vi "GUI_Frog_HPD_Version 2.0.vi"() -> ()   [LabVIEW 2020]
uses:
  Shared/GUI_Template/GUI_master/tcp_new_data_event.ctl
  Shared/GUI_Template/GUI_master/tcp new data cluster.ctl
  GUI_Cameras/color tables/image color table presets.ctl
  <vilib>/vision/Image Controls.llb/IMAQ Image.ctl
  <vilib>/vision/NI_Vision_Development_Module.lvlib
panel:
  in  "Color table":T1=enum."Binary"
  out "Time":sgl[](graph)
  out "Spectrum":sgl[](graph)
  out "tcp data event 2":T2
  out "Tank":dbl(slide) scale=0.0..255.0 scale format="%#_6p"
  out "131":T3(plugin-control) caption="Spatial Image"
  out "525":T3(plugin-control) caption="FROG Trace"
  out "error out":errorcluster
  in  "Clear":bool
  in  "UDP error message":string
  in  "Refresh Button":bool
  in  "Tab Control":T4(tab)
  in  "exposure::1":dbl=0.001 caption="Exposure" min=5.0 max=10000.0 format="%_4p"
  out "frogerrorfinal::1":dbl caption="Frog Error (<1% OK)" min=0.0 max=500.0
  in  "cameraselect::1":enum16{"temporal CAM", "spatial CAM"}(ring) caption="Select Camera"
  in  "triggermode::1":bool caption="Blank Button"
  in  "Select device":string(combo)="FrogHPD"
  out "GUIdevice 1":string="FrogHPD"
  out "element":string
  out "Application:Command Line Arguments":string[](array[string])
  out "max counts":cluster{dbl[], dbl[]}(graph)
  out "mean counts":cluster{dbl[], dbl[]}(graph)
  out "Fourier analyzed data":T5
  in  "fourier":bool
  out "SpatialImage::1":T3(plugin-control) caption="Spatial Image"
  out "frogTrace::1":T3(plugin-control) caption="FROG Trace"
  in  "insert tag":bool=TRUE
  in  "stop":bool
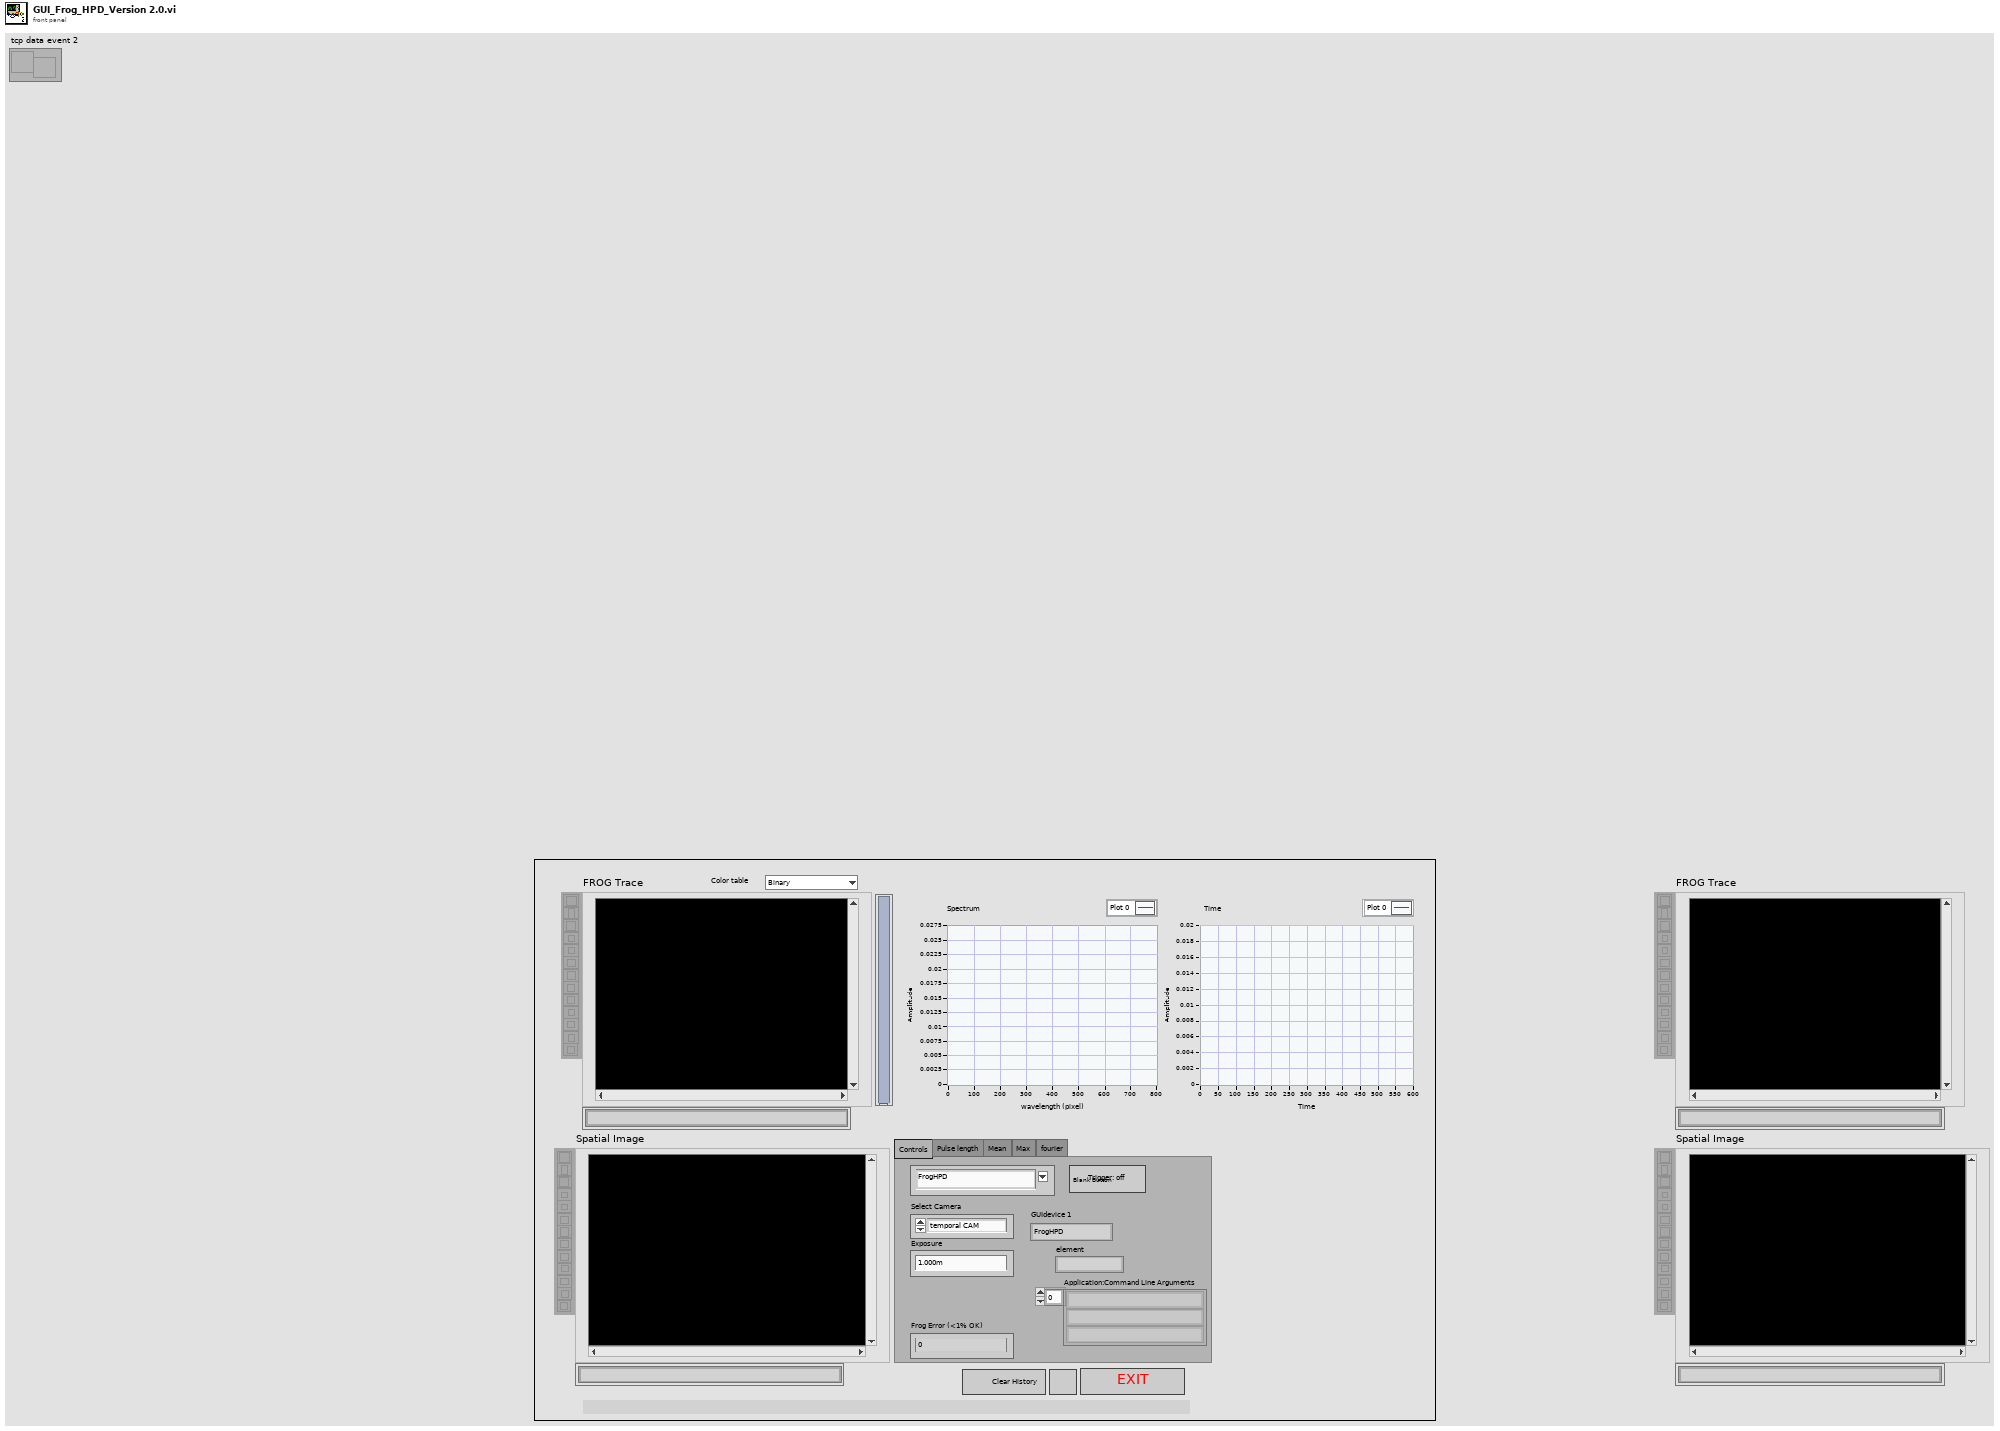
[diagram p1: front panel]
types:
  T1 = typedef "image color table presets.ctl" = enum16{"Greyscale", "Binary", "Gradient", "Rainbow", "Temperature", "enhance low", "blue yellow red", "BYR enhance low", "white blue yellow", "BWR enhance low", "make a new one"}
  T2 = typedef "tcp_new_data_event.ctl" = refnum<user-event>
  T3 = typedef "IMAQ Image.ctl" = refnum<image>
  T4 = enum32{"Controls", "Pulse length", "Mean", "Max", "fourier"}
  T5 = cluster{"Amplitude":dbl, "Frequency":dbl, "period":dbl}
  T6 = enum32{"invalid app kind", "Development System", "Run Time System", "Student Edition", "Embedded LabVIEW", "Evaluation", "Custom"}
  T7 = typedef "tcp new data cluster.ctl" = cluster{"EventEnum":enum16{"new data", "connection status update"}, "Device name":string}
  T8 = enum32{"Invalid", "Standard", "Closed", "Hidden", "Minimized", "Maximized"}
  T9 = cluster{"Left":i32, "Top":i32, "Right":i32, "Bottom":i32}
  T10 = cluster{"Core":cluster{"Current VI Reference":refnum<vi>, "Close Panel on Exit?":bool}, "Your Boolean data":bool, "Your string data":string, "SuperGUI":cluster{"STOP queue":refnum<queue>, "SuperGUI ref":refnum<vi>, "event reg":refnum<event-registration>}, "Images":cluster{"frogTrace::1":T3, "retrievedFrogTrace::1":T3, "SpatialImage::1":T3, "rotated_Temporal":T3, "rotated_Spatial":T3}}
  T11 = cluster{"frogTrace::1":T3, "retrievedFrogTrace::1":T3, "SpatialImage::1":T3, "rotated_Temporal":T3, "rotated_Spatial":T3}
  T12 = cluster{"STOP queue":refnum<queue>, "SuperGUI ref":refnum<vi>, "event reg":refnum<event-registration>}
  T13 = cluster{"Current VI Reference":refnum<vi>, "Close Panel on Exit?":bool}
  T14 = cluster{"histogram":u32[], "Minimal Value":sgl, "Maximal Value":sgl, "Starting Value":sgl, "Interval Width":sgl, "Mean Value":sgl, "Standard  Variation":sgl, "Area (pixels)":i32}
  T15 = typedef "Image Type" = u32
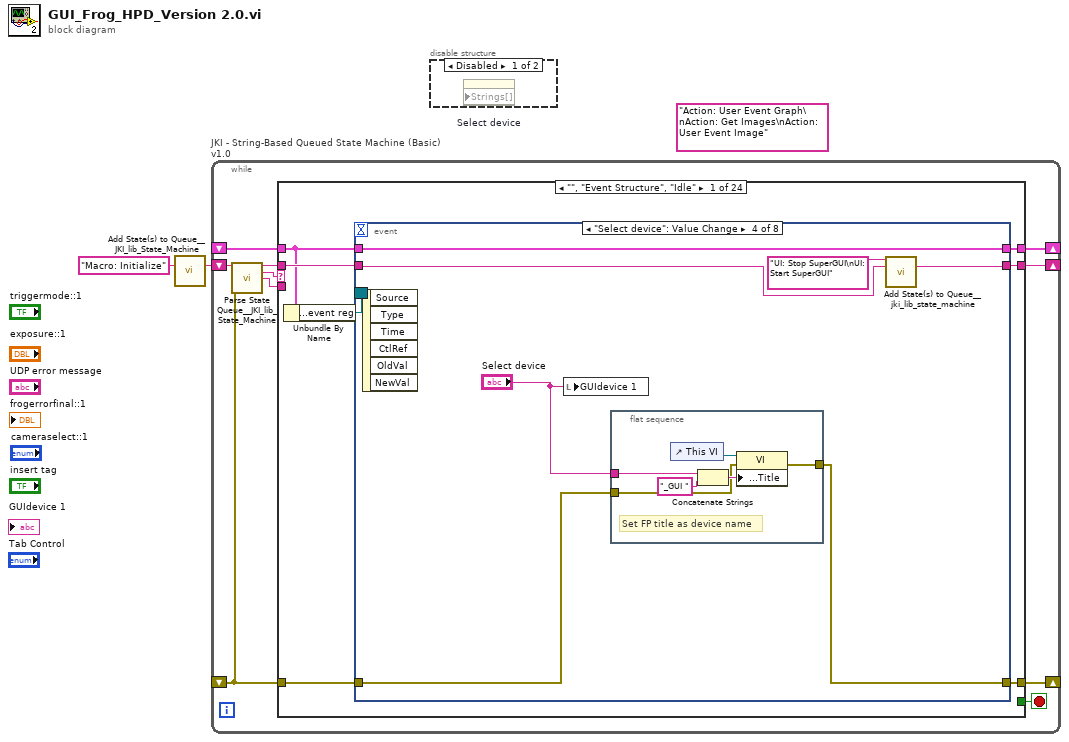
[diagram p0: block diagram]
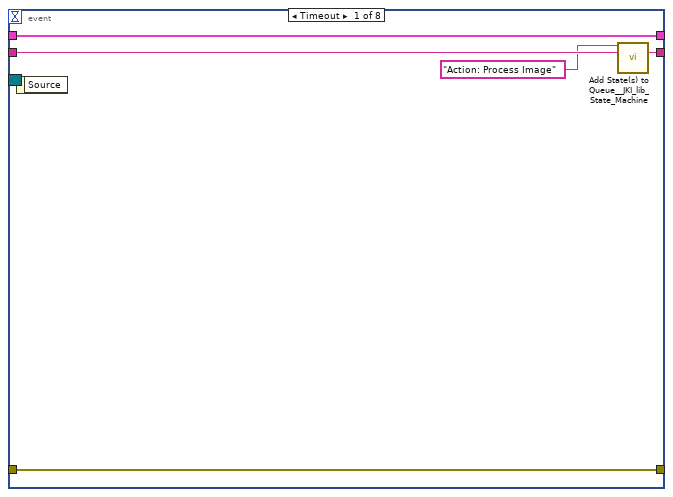
[diagram p3: hidden frame]
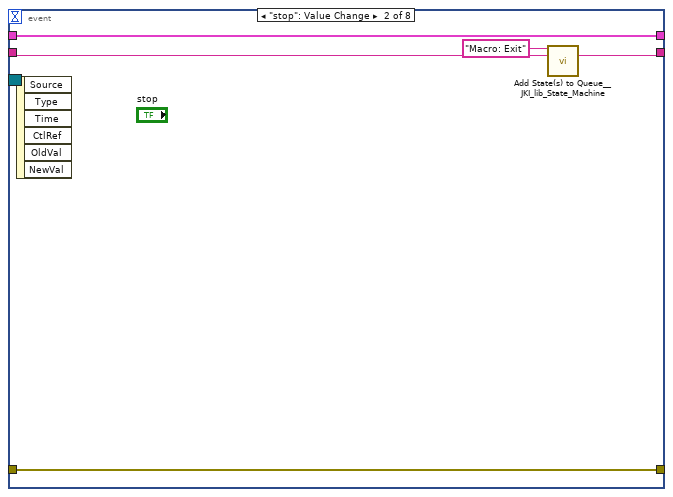
[diagram p4: hidden frame]
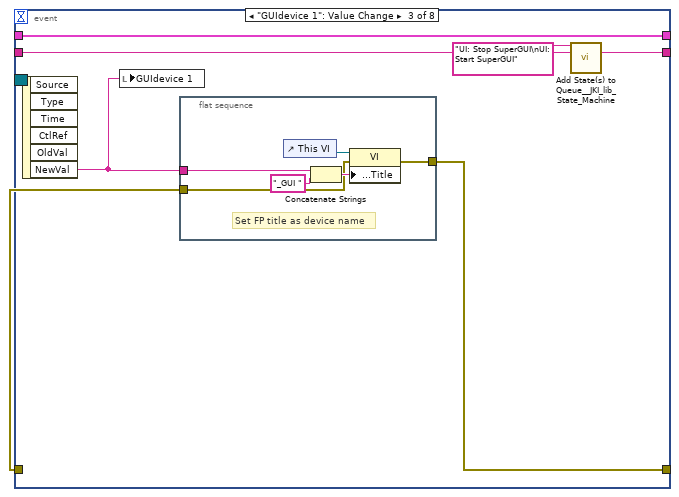
[diagram p5: hidden frame]
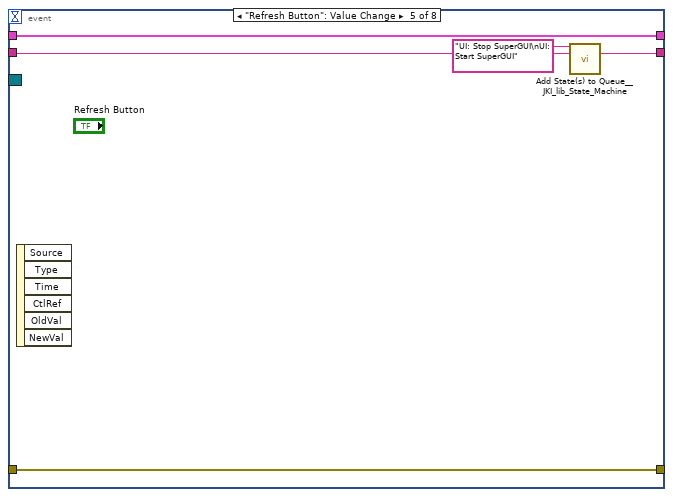
[diagram p6: hidden frame]
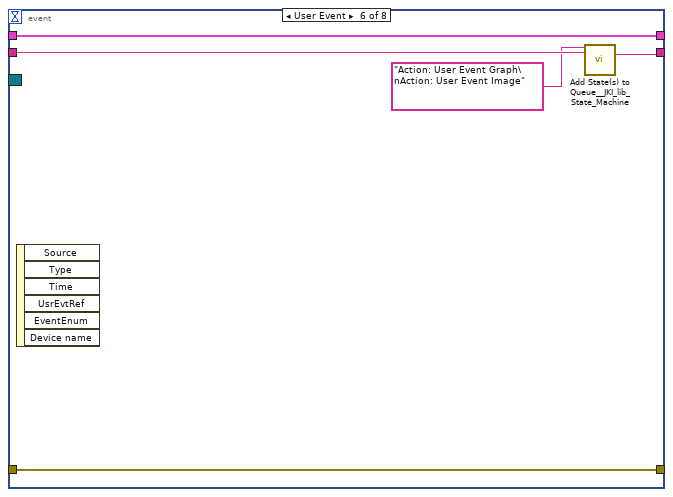
[diagram p7: hidden frame]
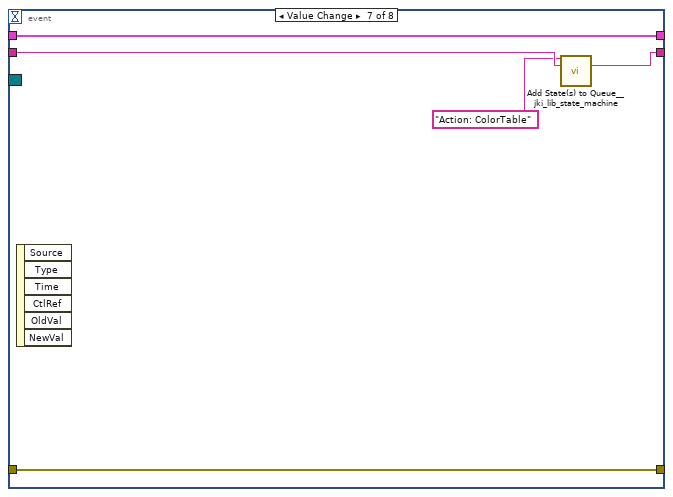
[diagram p8: hidden frame]
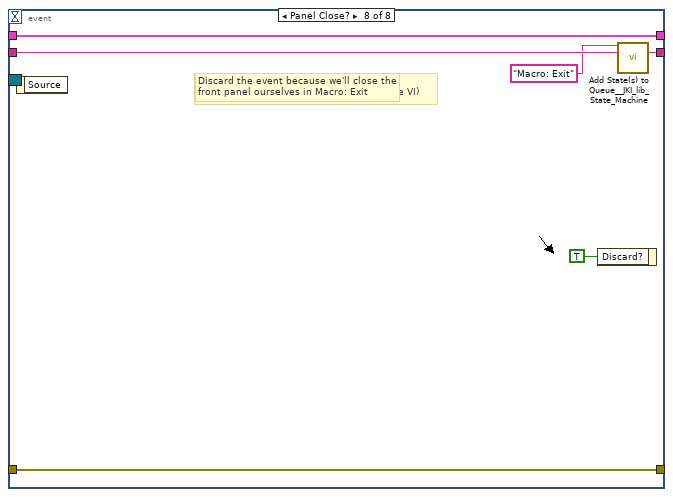
[diagram p9: hidden frame]
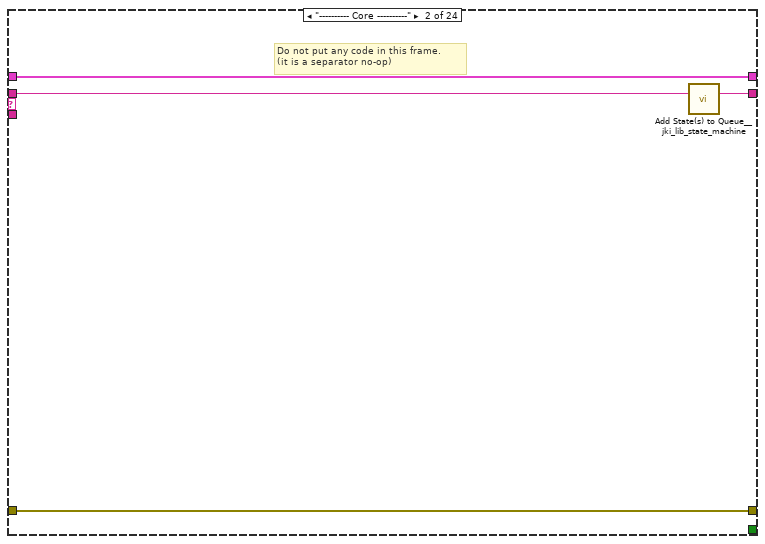
[diagram p10: hidden frame]
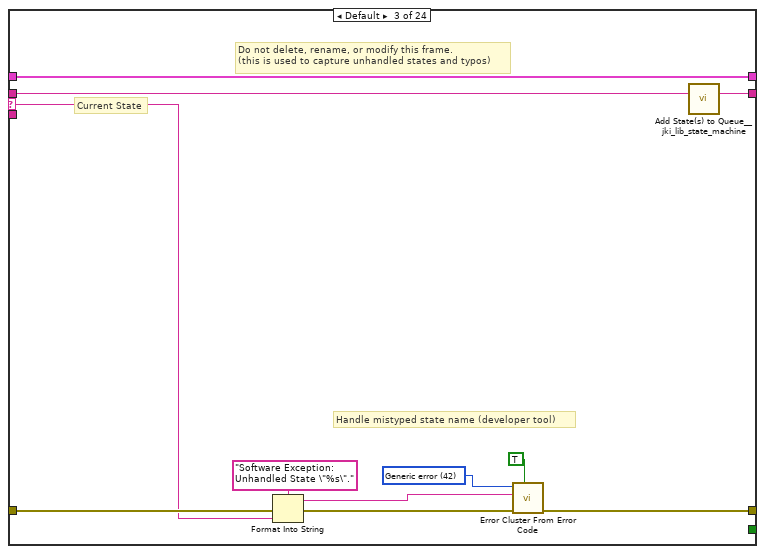
[diagram p11: hidden frame]
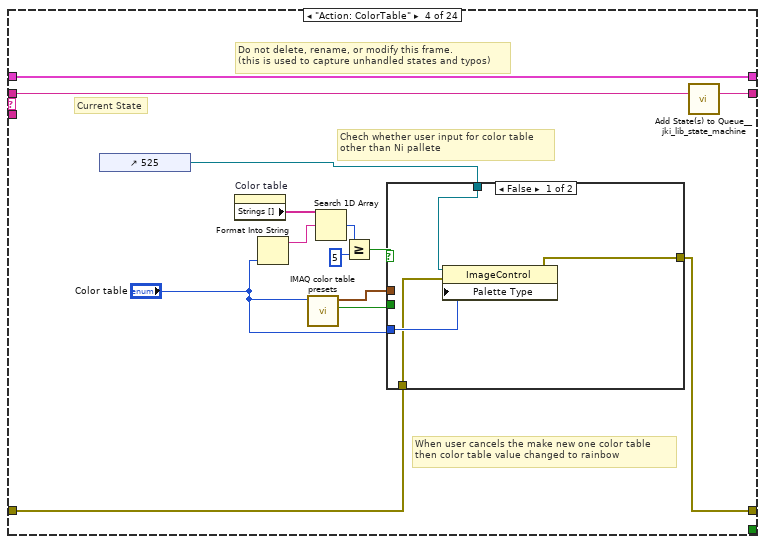
[diagram p12: hidden frame]
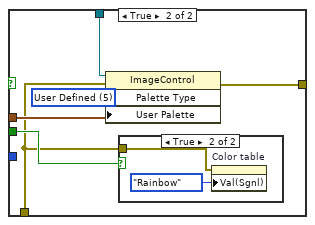
[diagram p13: hidden frame]
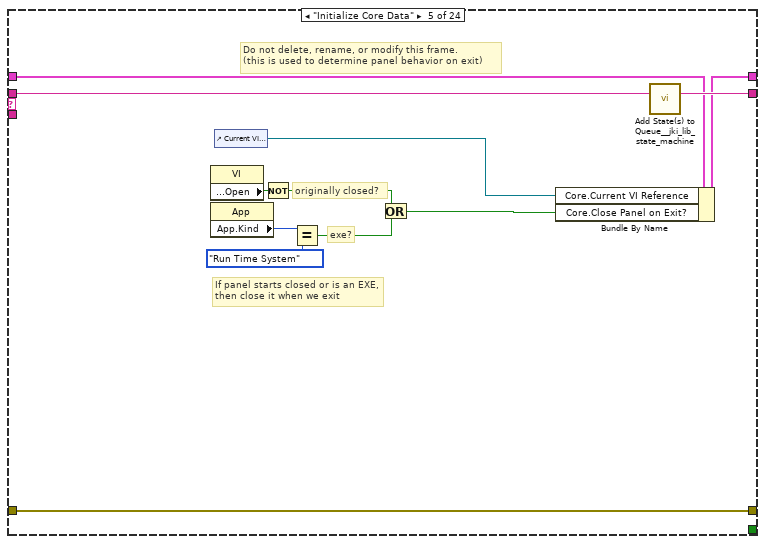
[diagram p15: hidden frame]
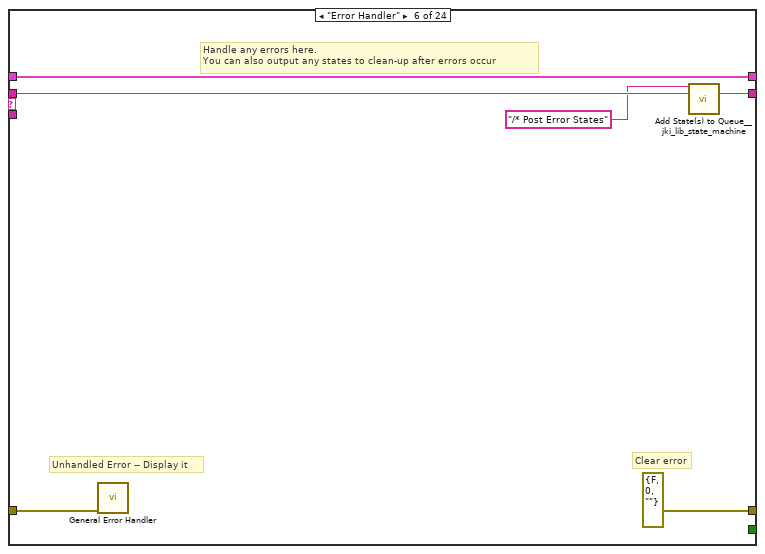
[diagram p16: hidden frame]
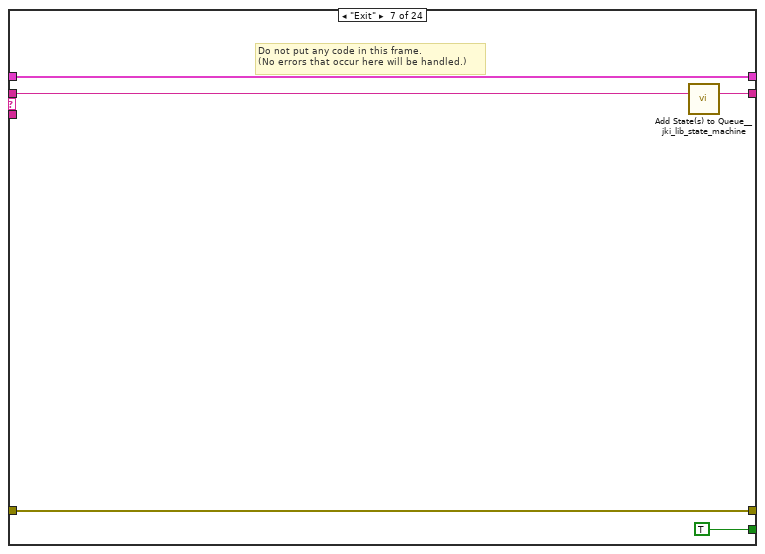
[diagram p17: hidden frame]
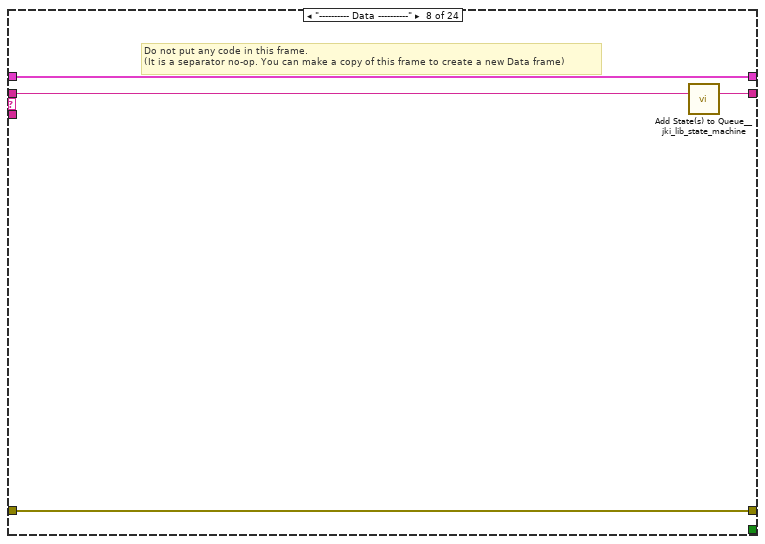
[diagram p18: hidden frame]
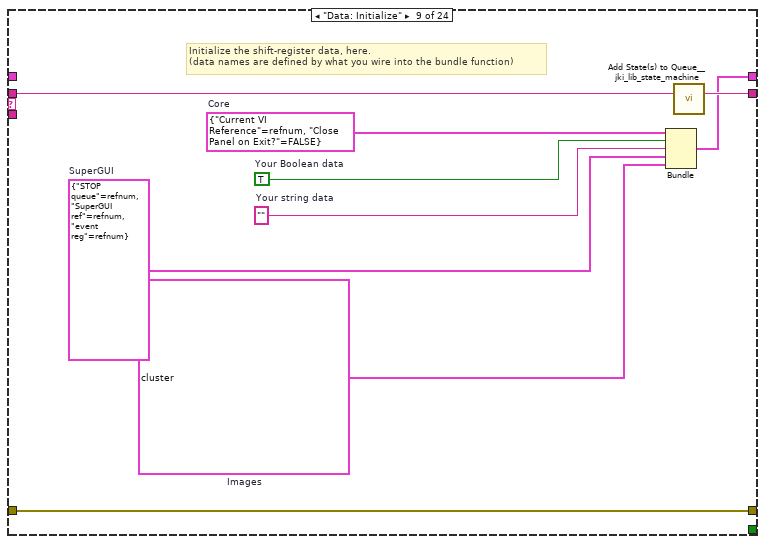
[diagram p19: hidden frame]
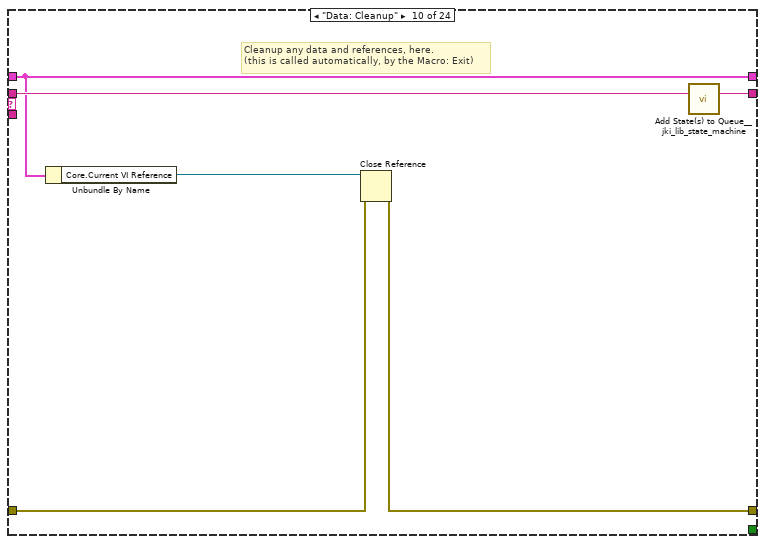
[diagram p20: hidden frame]
diagram:
  (unwired) "Action: User Event Graph\nAction: Get Images\nAction: User Event Image" ("State(s) in Front (\"\")")
  n1 = call <vilib>:"Add State(s) to Queue__JKI_lib_State_Machine.vi"("State(s) in (\"\")"="Macro: Initialize") -> ("States Out"=w2:string)  [unwired: 14 in]
  n2 = while "JKI - String-Based Queued State Machine (Basic) v1.0" {
    shift-right: [w5] -> _
    shift-left: _ -> [w4]
    shift-right: [w8] -> _
    shift-left: _ -> [w3]
    shift-right: [w7] -> _
    shift-left: w2 -> [w9]
    stop <- w6 stop-if-true
    n3 = call <vilib>:"Parse State Queue__JKI_lib_State_Machine.vi"("State Queue"=w9, "Error In (no error)"=w3) -> ("Remaining States"=w11:string, "Current State"=w12:string, "Arguments"=w10:string)  [unwired: 11 in]
    n4 = case shown="\"\", \"Event Structure\", \"Idle\"" w12 {
      selector: w12 -> [_ _ w81 _ _ _ _ _ _ _ _ _ _ _ _ _ _ _ _ _ _ _ _ _]
      tunnel: w11 -> [w19 w80 w85 w105 w129 w135 w140 w144 w153 w159 w163 w170 w176 w213 w221 w227 w238 w264 w269 w279 w283 w298 w318 w339]
      tunnel: w10 -> [_ _ _ _ _ _ _ _ _ _ _ _ _ _ _ w222 w232 _ _ _ _ _ _ _]
      tunnel: w4 -> [w14 w77 w83 w103 w120 w132 w138 w141 _ w154 w160 w168 w174 w204 w216 w225 w234 w261 w266 w276 w280 w295 w307 w323]
      tunnel: [w17 w78 w87 w93 w126 errorcluster {"status"=FALSE, "code"=0, "source"=""} ("error out") w137 w142 w150 w155 w161 w166 w171 w198 w214 w223 w235 w262 w267 w277 w281 w296 w316 w337] -> w8
      tunnel: w3 -> [w16 w78 w86 w94 w126 w131 w137 w142 w150 w156 w161 w167 w172 w199 w215 w224 w236 w262 w267 w277 w281 w296 w316 w337]
      tunnel: [w18 w79 w84 w104 w128 w134 w139 w143 w152 w158 w162 w169 w175 w212 w220 w226 w237 w263 w268 w278 w282 w297 w317 w338] -> w7
      tunnel: [_ _ _ _ _ _ TRUE _ _ _ _ _ _ _ _ _ _ _ _ _ _ _ _ _] -> w6
      tunnel: [w15 w77 w83 w103 w127 w132 w138 w141 w151 w154 w160 w168 w174 w203 w216 w225 w234 w261 w266 w276 w280 w295 w306 w323] -> w5
      frame "", "Event Structure", "Idle" {
        n5 = Unbundle By Name(w14) -> ("SuperGUI.event reg"=w13:refnum<event-registration>)
        n6 = event shown="[3] \"Select device\": Value Change" {
          selector: w13 -> [_ _ _ _ _ _ _ _]
          dyn-events: _ -> [_ _ _ _ _ _ _ _]
          timeout: _ -> [_ _ _ _ _ _ _ _]
          tunnel: w19 -> [w24 w27 w33 w45 w58 w64 w68 w76]
          tunnel: [w23 w26 w32 w44 w57 w63 w69 w75] -> w18
          tunnel: w14 -> [w21 w29 w36 w49 w60 w65 w70 w73]
          tunnel: [w22 w28 w34 w47 w59 w61 w66 w74] -> w17
          tunnel: w16 -> [w22 w28 w35 w48 w59 w61 w66 w74]
          tunnel: [w21 w29 w36 w49 w60 w65 w70 w73] -> w15
          event Timeout {
            n7 = event-data() -> ()  [unwired: 1 in, 1 out]
            n8 = call <vilib>:"Add State(s) to Queue__JKI_lib_State_Machine.vi"("State(s) in Front (\"\")"="Action: Process Image" ("State(s) in Front (\"\")"), "State(s) in (\"\")"=w24) -> ("States Out"=w23:string)  [unwired: 13 in]
          }
          event "stop": Value Change {
            n9 = event-data() -> ()  [unwired: 1 in, 6 out]
            n10 = call <vilib>:"Add State(s) to Queue__JKI_lib_State_Machine.vi"("State(s) in Front (\"\")"="Macro: Exit", "State(s) in (\"\")"=w27) -> ("States Out"=w26:string)  [unwired: 13 in]
          }
          event "GUIdevice 1": Value Change {
            n11 = event-data() -> ("NewVal"=w30:string)  [unwired: 1 in, 5 out]
            n12 = local write "GUIdevice 1"(w30) -> ()
            n13 = flat-sequence {
              tunnel: [w39] -> w34
              tunnel: w35 -> [w38]
              tunnel: w30 -> [w37]
              frame #0 {
                # "Set FP title as device name"
                n14 = control-ref of="This VI"() -> (w42:refnum<vi>)
                n15 = Concatenate Strings(w37, "_GUI ") -> (w41:string)
                n16 = property class="VI"(reference=w42, error in=w38, "Front Panel.Title"=w41) -> (error out=w39:errorcluster)  [unwired: 1 out]
              }
            }
            n17 = call <vilib>:"Add State(s) to Queue__JKI_lib_State_Machine.vi"("State(s) in Front (\"\")"="UI: Stop SuperGUI\nUI: Start SuperGUI", "State(s) in (\"\")"=w33) -> ("States Out"=w32:string)  [unwired: 13 in]
          }
          event "Select device": Value Change {
            n18 = event-data() -> ()  [unwired: 1 in, 6 out]
            n19 = local write "GUIdevice 1"("Select device") -> ()
            n20 = flat-sequence {
              tunnel: [w52] -> w47
              tunnel: w48 -> [w51]
              tunnel: "Select device" -> [w50]
              frame #0 {
                # "Set FP title as device name"
                n21 = control-ref of="This VI"() -> (w55:refnum<vi>)
                n22 = Concatenate Strings(w50, "_GUI ") -> (w54:string)
                n23 = property class="VI"(reference=w55, error in=w51, "Front Panel.Title"=w54) -> (error out=w52:errorcluster)  [unwired: 1 out]
              }
            }
            n24 = call <vilib>:"Add State(s) to Queue__jki_lib_state_machine.vi"("State(s) in Front (\"\")"="UI: Stop SuperGUI\nUI: Start SuperGUI", "State(s) in (\"\")"=w45) -> ("States Out"=w44:string)  [unwired: 13 in]
          }
          event "Refresh Button": Value Change {
            n25 = event-data() -> ()  [unwired: 1 in, 6 out]
            n26 = call <vilib>:"Add State(s) to Queue__JKI_lib_State_Machine.vi"("State(s) in Front (\"\")"="UI: Stop SuperGUI\nUI: Start SuperGUI", "State(s) in (\"\")"=w58) -> ("States Out"=w57:string)  [unwired: 13 in]
          }
          event User Event {
            n27 = event-data() -> ()  [unwired: 1 in, 6 out]
            n28 = call <vilib>:"Add State(s) to Queue__JKI_lib_State_Machine.vi"("State(s) in Front (\"\")"="Action: User Event Graph\nAction: User Event Image" ("State(s) in Front (\"\")"), "State(s) in (\"\")"=w64) -> ("States Out"=w63:string)  [unwired: 13 in]
          }
          event Value Change {
            n29 = event-data() -> ()  [unwired: 1 in, 6 out]
            n30 = call <vilib>:"Add State(s) to Queue__jki_lib_state_machine.vi"("State(s) in Front (\"\")"="Action: ColorTable" ("State(s) in Front (\"\")"), "State(s) in (\"\")"=w68) -> ("States Out"=w69:string)  [unwired: 13 in]
          }
          event Panel Close? {
            # "Discard the event because we'll close the front panel ourselves in Macro: Exit"
            # "Close Panel button (pressed) Event\n(this executes Macro: Exit to terminate the VI)"
            n31 = event-data() -> ()  [unwired: 1 in, 1 out]
            n32 = event-data("Discard?"=TRUE) -> ()  [unwired: 1 in, 1 out]
            n33 = call <vilib>:"Add State(s) to Queue__JKI_lib_State_Machine.vi"("State(s) in Front (\"\")"="Macro: Exit", "State(s) in (\"\")"=w76) -> ("States Out"=w75:string)  [unwired: 13 in]
          }
        }
      }
      frame "---------- Core ----------" {
        # "Do not put any code in this frame.\n(it is a separator no-op)"
        n34 = call <vilib>:"Add State(s) to Queue__jki_lib_state_machine.vi"("State(s) in (\"\")"=w80) -> ("States Out"=w79:string)  [unwired: 14 in]
      }
      frame Default {
        w90 = 42 items=["No error", "Argument error", "Memory is full", "Out of zone", "End of file", "File already open", "Generic file I/O error", "File not found", "File permission error", "Disk is full", "Duplicate path", "Too many files open", "System feature not enabled", "Resource file not found", "Cannot add resource", "Resource not found", "Image not found", "Image memory error", "Pen does not exist", "Config type invalid", "Config token not found", "Config parse error", "Config memory error", "Bad external code format", "Bad external code offset", "External code not present", "Null window", "Destroy window error", "Null menu", "Print aborted", "Bad print record", "Print driver error", "Windows error during printing", "Memory error during printing", "Print dialog error", "Generic print error", "Invalid device refnum", "Device not found", "Device parameter error", "Device unit error", "Cannot open device", "Device call aborted", "Generic error", "Cancelled by user", "Object ID too low", "Object ID too high", "Object not in heap", "Unknown heap", "Unknown object (invalid DefProc)", "Unknown object (DefProc not in table)", "Message out of range", "Invalid (null) method", "Unknown message", "Manager call not supported", "Bad address", "Network operation in progress", "Network operation timed out", "Connection is busy", "Network attribute not supported", "Network error", "Address in use", "System out of memory", "Connection aborted", "Connection refused", "Not connected", "Already connected", "Connection closed", "Initialization error (interapplication manager)", "Bad occurrence", "Wait on unbound occurrence handler", "Occurrence queue overflow", "Datalog type conflict", "Unused", "Unrecognized type (interapplication manager)", "Memory corrupt", "Failed to make temporary DLL", "Old CIN version", "Drag socket not found", "Failed to load drop-object", "Failed to register OLE object", "Failed to release OLE object", "Format specifier type mismatch", "Unknown format specifier", "Too few format specifiers", "Too many format specifiers", "Scan failed", "Newer CIN version", "Error converting to variant", "Runtime menu error", "Password tampered", "Variant attribute not found", "Incompatible variant data type", "Event data is not available", "Event Store is not present", "Occurrence is not found", "Event Queue is not created", "Event info is not available", "Refnum passed is NULL", "Error retrieving Class GUID", "Error retrieving CoClass GUID", "Error retrieving TypeLib GUID.", "Bad built application magic bytes.", "Specific driver is different from the specific driver associated with the Logical Name.", "There is no session opened to the class driver.", "Max Error", "MAX - Error with config objects", "MAX - Error loading configuration", "MAX - Group not supported"]
        # "Current State"
        # "Do not delete, rename, or modify this frame.\n(this is used to capture unhandled states and typos)"
        # "Handle mistyped state name (developer tool)"
        n35 = Format Into String(format string="Software Exception: Unhandled State \"%s\"." ("message"), error in=w86, w81) -> (resulting string=w89:string, error out=w88:errorcluster)  [unwired: 1 in]
        n36 = call <vilib>:"Error Cluster From Error Code.vi"("show call chain? (False)"=TRUE, "error in (no error)"=w88, "error message (\"\")"=w89, "error code (0)"=w90) -> ("error out"=w87:errorcluster)  [unwired: 5 in]
        n37 = call <vilib>:"Add State(s) to Queue__jki_lib_state_machine.vi"("State(s) in (\"\")"=w85) -> ("States Out"=w84:string)  [unwired: 14 in]
      }
      frame "Action: ColorTable" {
        # "Chech whether user input for color table\nother than Ni pallete"
        # "When user cancels the make new one color table \nthen color table value changed to rainbow"
        # "Current State"
        # "Do not delete, rename, or modify this frame.\n(this is used to capture unhandled states and typos)"
        n38 = control-ref of="525"() -> (w92:refnum<vi>)
        n39 = property on="Color table" class="Enum (strict)"() -> ("Strings []"=w99:string[])  [unwired: 2 in, 2 out]
        n40 = Format Into String("Color table") -> (resulting string=w100:string)  [unwired: 3 in, 1 out]
        n41 = call "IMAQ color table presets.vi"("Color table"="Color table") -> ("Make new one cancelled"=w95:bool, "Array"=w102:cluster{"R":u8, "G":u8, "B":u8}[])  [unwired: 9 in]
        n42 = Search 1D Array(1D array=w99, element=w100) -> (index of element=w97:i32)  [unwired: 1 in]
        n43 = Greater Or Equal?(x=w97, y=5) -> (x >= y?=w98:bool)
        n44 = case shown="False" w98 {
          tunnel: w102 -> [_ w114]
          tunnel: "Color table" -> [w109 _]
          tunnel: w94 -> [w108 w111]
          tunnel: [w107 w113] -> w93
          tunnel: w95 -> [_ w112]
          tunnel: w92 -> [w106 w110]
          frame False {
            n45 = property on="Property Node" class="ImageControl"(reference=w106, error in=w108, "Palette Type"=w109) -> (error out=w107:errorcluster)  [unwired: 1 out]
          }
          frame True {
            w115 = u32 5 items=["Grayscale", "Binary", "Gradient", "Rainbow", "Temperature", "User Defined"] ("Palette:Palette Type")
            n46 = property on="Property Node" class="ImageControl"(reference=w110, error in=w111, "Palette Type"=w115, "User Palette"=w114) -> (error out=w113:errorcluster)  [unwired: 1 out]
            n47 = case shown="True" w112 {
              tunnel: w111 -> [_ w116]
              frame False {
              }
              frame True {
                n48 = property on="Color table" class="Enum (strict)"(error in=w116, "Val(Sgnl)"=image_color_table_presets."Rainbow" ("Value (Signaling)")) -> ()  [unwired: 1 in, 2 out]
              }
            }
          }
        }
        n49 = call <vilib>:"Add State(s) to Queue__jki_lib_state_machine.vi"("State(s) in (\"\")"=w105) -> ("States Out"=w104:string)  [unwired: 14 in]
      }
      frame "Initialize Core Data" {
        # "Do not delete, rename, or modify this frame.\n(this is used to determine panel behavior on exit)"
        # "originally closed?"
        # "exe?"
        # "If panel starts closed or is an EXE, then close it when we exit"
        n50 = property class="VI"() -> ("Front Panel.Open"=w125:bool)  [unwired: 2 in, 2 out]
        n51 = property class="App"() -> ("App.Kind"=w124:T6)  [unwired: 2 in, 2 out]
        n52 = control-ref of="Current VI Reference"() -> (w118:refnum<vi>)
        n53 = Not(x=w125) -> (.not. x?=w122:bool)
        n54 = Equal?(x=w124, y=T6."Run Time System" ("Application:Kind")) -> (x = y?=w121:bool)
        n55 = Or(x=w122, y=w121) -> (x .or. y?=w119:bool)
        n56 = Bundle By Name(cluster=w120, "Core.Current VI Reference"=w118, "Core.Close Panel on Exit?"=w119) -> (w127:T10)
        n57 = call <vilib>:"Add State(s) to Queue__jki_lib_state_machine.vi"("State(s) in (\"\")"=w129) -> ("States Out"=w128:string)  [unwired: 14 in]
      }
      frame "Error Handler" {
        # "Unhandled Error -- Display it"
        # "Handle any errors here.\nYou can also output any states to clean-up after errors occur"
        # "Clear error"
        n58 = call <vilib>:"General Error Handler.vi"("error in (no error)"=w131) -> ()  [unwired: 10 in, 5 out]
        n59 = call <vilib>:"Add State(s) to Queue__jki_lib_state_machine.vi"("State(s) in Front (\"\")"="/* Post Error States", "State(s) in (\"\")"=w135) -> ("States Out"=w134:string)  [unwired: 13 in]
      }
      frame "Exit" {
        # "Do not put any code in this frame.\n(No errors that occur here will be handled.)"
        n60 = call <vilib>:"Add State(s) to Queue__jki_lib_state_machine.vi"("State(s) in (\"\")"=w140) -> ("States Out"=w139:string)  [unwired: 14 in]
      }
      frame "---------- Data ----------" {
        # "Do not put any code in this frame.\n(It is a separator no-op. You can make a copy of this frame to create a new Data frame)"
        n61 = call <vilib>:"Add State(s) to Queue__jki_lib_state_machine.vi"("State(s) in (\"\")"=w144) -> ("States Out"=w143:string)  [unwired: 14 in]
      }
      frame "Data: Initialize" {
        w145 = T11 {"frogTrace::1"="remote image 000000001D2B938C", "retrievedFrogTrace::1"="remote image 000000001D2B938C", "SpatialImage::1"="remote image 000000001D2B938C", "rotated_Temporal"=refnum, "rotated_Spatial"=refnum}  # Images
        w146 = T12 {"STOP queue"=refnum, "SuperGUI ref"=refnum, "event reg"=refnum}  # SuperGUI
        w147 = T13 {"Current VI Reference"=refnum, "Close Panel on Exit?"=FALSE}  # Core
        w149 = TRUE  # Your Boolean data
        w148 = ""  # Your string data
        # "Initialize the shift-register data, here.\n(data names are defined by what you wire into the bundle function)"
        n62 = Bundle("Core"=w147, "Your Boolean data"=w149, "Your string data"=w148, "SuperGUI"=w146, "Images"=w145) -> (w151:T10)  [unwired: 1 in]
        n63 = call <vilib>:"Add State(s) to Queue__jki_lib_state_machine.vi"("State(s) in (\"\")"=w153) -> ("States Out"=w152:string)  [unwired: 14 in]
      }
      frame "Data: Cleanup" {
        # "Cleanup any data and references, here.\n(this is called automatically, by the Macro: Exit)"
        n64 = Unbundle By Name(w154) -> ("Core.Current VI Reference"=w157:refnum<vi>)
        n65 = Close Reference(reference=w157, error in (no error)=w156) -> (error out=w155:errorcluster)
        n66 = call <vilib>:"Add State(s) to Queue__jki_lib_state_machine.vi"("State(s) in (\"\")"=w159) -> ("States Out"=w158:string)  [unwired: 14 in]
      }
      frame "---------- UI ----------" {
        # "Do not put any code in this frame.\n(It is a separator no-op. You can make a copy of this frame to create a new UI frame)"
        n67 = call <vilib>:"Add State(s) to Queue__jki_lib_state_machine.vi"("State(s) in (\"\")"=w163) -> ("States Out"=w162:string)  [unwired: 14 in]
      }
      frame "UI: Initialize" {
        # "Initialize the User Interface, here.\n(this is called automatically, by the Macro: Init)"
        n68 = call <userlib>:"Fit VI window to Largest Dec__ogtk.vi"("error in (no error)"=w167) -> ("error out"=w166:errorcluster)  [unwired: 5 in, 1 out]
        n69 = call "getDevices.vi"("Device Class"="FROG") -> ("All Devices"=w164:string[])  [unwired: 1 out]
        n70 = property on="Select device" class="CmbBox"("Strings[]"=w164) -> ()  [unwired: 2 in, 2 out]
        n71 = call <vilib>:"Add State(s) to Queue__jki_lib_state_machine.vi"("State(s) in (\"\")"=w170) -> ("States Out"=w169:string)  [unwired: 14 in]
      }
      frame "UI: Get Device Name" {
        # "Initialize the User Interface, here.\n(this is called automatically, by the Macro: Init)"
        n72 = First Call?() -> (First Call?: T/F=w173:bool)
        n73 = case shown="True" w173 {
          tunnel: w172 -> [w177 w179]
          tunnel: [w177 w178] -> w171
          frame False {
          }
          frame True {
            n74 = disable-structure "Get Device name from control for vi mode\nand command line arg for exe" shown="RUN_TIME_ENGINE==True" {
              disable-tunnel: w179 -> [w180 w183]
              disable-tunnel: [w180 w182] -> w178
              frame condition #0 (active) {
              }
              frame condition #1 {
                n75 = control-ref of="This Application"() -> (w181:refnum<vi>)
                n76 = property class="App"(reference=w181) -> ("App.Args"=w190:string[])  [unwired: 1 in, 2 out]
                "Application:Command Line Arguments" <- w190
                n77 = Index Array(array=w190, index #1=1 ("index")) -> (element #1=w184:string)  [unwired: 2 in, 2 out]
                "element" <- w184
                n78 = Empty String/Path?(string/path=w184) -> (empty?=w188:bool)
                n79 = control-ref of="This VI"() -> (w187:refnum<vi>)
                n80 = case shown="False" w188 {
                  tunnel: w184 -> [w191 _]
                  frame False {
                    n81 = local write "GUIdevice 1"(w191) -> ()
                    n82 = local write "Select device"(w191) -> ()
                  }
                  frame True {
                  }
                }
                n83 = Concatenate Strings(w184, "_GUI ") -> (w186:string)
                n84 = property class="VI"(reference=w187, error in=w183, "Front Panel.Title"=w186) -> (error out=w182:errorcluster)  [unwired: 1 out]
              }
            }
          }
        }
        n85 = call <vilib>:"Add State(s) to Queue__jki_lib_state_machine.vi"("State(s) in (\"\")"=w176) -> ("States Out"=w175:string)  [unwired: 14 in]
      }
      frame "UI: Start SuperGUI" {
        # "create stop queue for supergui and its clones"
        # "x100 abort will be dependent on caller VI\nx80 abort will be independent of caller vi, this will abort vi when labview is closed."
        # "Start SuperGUI asynchronous way"
        n86 = vi-ref "GUI_Master_subvi_reentrant_queues.vi"() -> (w197:refnum<vi>)
        n87 = property class="VI"(reference=w197) -> ("Path"=w196:path)  [unwired: 1 in, 2 out]
        n88 = Create User Event(user event datatype=T7 {"EventEnum"=enum."new data", "Device name"="Device name"} ("New Event"), error in=w199) -> (user event=w194:refnum<user-event>, error out=w205:errorcluster)
        "tcp data event 2" <- w194
        n89 = control-ref of="This Application"() -> (w202:refnum<vi>)
        n90 = control-ref of="This VI"() -> (w201:refnum<vi>)
        n91 = Open VI Reference(type specifier VI Refnum (for type only)=refnum<vi> refnum, vi path=w196, options=256) -> (vi reference=w211:refnum<vi>, error out=w210:errorcluster)  [unwired: 3 in]
        n92 = register-events(w194) -> (reference out=w193:refnum<event-registration>)  [unwired: 2 in, 1 out]
        n93 = call "supergui create stop queue.vi"() -> ("STOP Queue out"=w207:refnum<queue>)  [unwired: 11 in]
        n94 = Current VI's Menubar() -> (w200:refnum<k9>)
        n95 = call-by-ref "Start Asynchronous Call"(reference=w211, error in=w210, "STOP Queue in"=w207, "This Application"=w202, 8:"error in (no error)"=w205, "tcp data event"=w194, "Caller menu reference"=w200, "Caller VI ref"=w201) -> (reference out=w195:refnum<vi>, error out=w198:errorcluster)  [unwired: 5 in, 1 out]
        n96 = Bundle By Name(cluster=w204, "SuperGUI.event reg"=w193, "SuperGUI.SuperGUI ref"=w195, "SuperGUI.STOP queue"=w207) -> (w203:T10)
        n97 = call <vilib>:"Add State(s) to Queue__jki_lib_state_machine.vi"("State(s) in Front (\"\")"="Action: Get Images" ("State(s) in Front (\"\")"), "State(s) in (\"\")"=w213) -> ("States Out"=w212:string)  [unwired: 13 in]
      }
      frame "UI: Stop SuperGUI" {
        # "Stop Supergui Clone and wait until it exit properly"
        n98 = Unbundle By Name(w216) -> ("SuperGUI.SuperGUI ref"=w218:refnum<vi>, "SuperGUI.STOP queue"=w217:refnum<queue>)
        n99 = Release Queue(queue=w217, error in (no error)=w215) -> (error out=w219:errorcluster)  [unwired: 1 in, 2 out]
        n100 = call-by-ref "Wait On Asynchronous Call"(reference=w218, error in=w219) -> ("error out"=w214:errorcluster)  [unwired: 11 in, 2 out]
        n101 = call <vilib>:"Add State(s) to Queue__jki_lib_state_machine.vi"("State(s) in (\"\")"=w221) -> ("States Out"=w220:string)  [unwired: 14 in]
      }
      frame "UI: Cursor Set" {
        # "Argument"
        # "Set and Unset Cursor Busy.\n(Usage: \"UI: Cursor Set >> Busy|Idle\")"
        n102 = case shown="\"Idle\", Default" w222 {
          tunnel: w224 -> [w229 w231]
          tunnel: [w228 w230] -> w223
          frame "Idle", Default {
            n103 = call <vilib>:"Unset Busy.vi"("error in (no error)"=w229) -> ("error out"=w228:errorcluster)  [unwired: 10 in]
          }
          frame "Busy" {
            n104 = call <vilib>:"Set Busy.vi"("error in (no error)"=w231) -> ("error out"=w230:errorcluster)  [unwired: 9 in, 1 out]
          }
        }
        n105 = call <vilib>:"Add State(s) to Queue__jki_lib_state_machine.vi"("State(s) in (\"\")"=w227) -> ("States Out"=w226:string)  [unwired: 14 in]
      }
      frame "UI: Front Panel State" {
        # "Argument"
        # "Set Front Panel Open or Closed\n(Usage: \"UI: Front Panel State >> Open|Close\")"
        n106 = Unbundle By Name(w234) -> ("Core.Current VI Reference"=w233:refnum<vi>)
        n107 = case shown="\"Open\", Default" w232 {
          tunnel: w236 -> [w242 w255]
          tunnel: [w244 w256] -> w235
          tunnel: w233 -> [w243 w253]
          frame "Open", Default {
            n108 = property class="VI"(reference=w243, error in=w242) -> (reference out=w240:refnum<vi>, error out=w241:errorcluster, "Front Panel.Open"=w239:bool)
            n109 = case shown="False" w239 {
              tunnel: [w247 w250] -> w244
              tunnel: w241 -> [w246 w250]
              tunnel: w240 -> [w245 _]
              frame False {
                n110 = invoke class="VI" method="FP.Open"(reference=w245, error in=w246, "Activate"=TRUE, "State"=T8."Standard") -> (error out=w247:errorcluster)  [unwired: 1 in, 4 out]
              }
              frame True {
              }
            }
          }
          frame "Close" {
            n111 = property class="VI"(reference=w253, error in=w255) -> (reference out=w252:refnum<vi>, error out=w254:errorcluster, "Front Panel.Open"=w251:bool)
            n112 = case shown="True" w251 {
              tunnel: [w257 w260] -> w256
              tunnel: w254 -> [w257 w259]
              tunnel: w252 -> [_ w258]
              frame False {
              }
              frame True {
                n113 = invoke class="VI" method="FP.Close"(reference=w258, error in=w259) -> (error out=w260:errorcluster)  [unwired: 1 in, 2 out]
              }
            }
          }
        }
        n114 = call <vilib>:"Add State(s) to Queue__jki_lib_state_machine.vi"("State(s) in (\"\")"=w238) -> ("States Out"=w237:string)  [unwired: 14 in]
      }
      frame "---------- Macro ----------" {
        # "Do not put any code in this frame.\n(It is a separator no-op. You can make a copy of this frame to create a new Macro frame)"
        n115 = call <vilib>:"Add State(s) to Queue__jki_lib_state_machine.vi"("State(s) in (\"\")"=w264) -> ("States Out"=w263:string)  [unwired: 14 in]
      }
      frame "Macro: Initialize" {
        # "Initialization Macro\n(This is called once, when the VI starts)"
        n116 = call <vilib>:"Add State(s) to Queue__jki_lib_state_machine.vi"("State(s) in Front (\"\")"="Data: Initialize\nInitialize Core Data\nUI: Initialize\nUI: Get Device Name\nUI: Start SuperGUI\nUI: Front Panel State >> Open", "State(s) in (\"\")"=w269) -> ("States Out"=w268:string)  [unwired: 13 in]
      }
      frame "Macro: Exit" {
        # "Exit Macro\n(This is called once, when the VI exits)"
        n117 = Unbundle By Name(w276) -> ("Core.Close Panel on Exit?"=w275:bool)
        n118 = Select(t="UI: Front Panel State >> Close", s=w275, f="") -> (s? t:f=w272:string)
        n119 = call <vilib>:"Add State(s) to Queue__jki_lib_state_machine.vi"("State(s) in (\"\")"=w272, "State(s) at Back (\"\")"="Data: Cleanup\nExit") -> ("States Out"=w270:string)  [unwired: 13 in]
        n120 = call <vilib>:"Add State(s) to Queue__jki_lib_state_machine.vi"("State(s) in Front (\"\")"=w270, "State(s) in (\"\")"=w279) -> ("States Out"=w278:string)  [unwired: 13 in]
      }
      frame "---------- New Category ----------" {
        # "Template Separator\n(You can make a copy of, or modify, this frame)"
        n121 = call <vilib>:"Add State(s) to Queue__jki_lib_state_machine.vi"("State(s) in (\"\")"=w283) -> ("States Out"=w282:string)  [unwired: 14 in]
      }
      frame "Action: User Event Graph" {
        w292 = 1000 ("max points")
        n122 = local read "frogTrace::1"() -> (w286:T3)
        n123 = call "IMAQ Histogram"("Image"=w286) -> ("Histogram Report"=w287:T14)  [unwired: 9 in, 1 out]
        n124 = call "IMAQ LinearAverages"("Image Src"=w286) -> ("Y Axis Averages"=→"Time":sgl[], "X Axis Averages"=→"Spectrum":sgl[])  [unwired: 6 in, 3 out]
        n125 = Unbundle By Name(w287) -> ("Maximal Value"=w288:sgl, "Mean Value"=w289:sgl)
        n126 = case shown="False" "Clear" {
          frame False {
          }
          frame True {
            n127 = local write "Clear"(FALSE ("Clear")) -> ()
          }
        }
        n128 = call "add value to xy graph.vi"("new value"=w288, "max points"=w292, "Wire in Stop To Clear Graph on Each Run"="Clear") -> ("XY Graph"=w293:cluster{dbl[], dbl[]})  [unwired: 8 in]
        "max counts" <- w293
        n129 = call "add value to xy graph.vi"("new value"=w289, "max points"=w292, "Wire in Stop To Clear Graph on Each Run"="Clear") -> ("XY Graph"=→"mean counts":cluster{dbl[], dbl[]})  [unwired: 8 in]
        n130 = case shown="True" "fourier" {
          tunnel: w293 -> [_ w300]
          frame False {
          }
          frame True {
            n131 = call "fourier analysis xy graph.vi"("xy graph"=w300) -> ("Fourier analyzed data"=→"Fourier analyzed data":T5)  [unwired: 9 in, 1 out]
          }
        }
        n132 = call <vilib>:"Add State(s) to Queue__jki_lib_state_machine.vi"("State(s) in (\"\")"=w298) -> ("States Out"=w297:string)  [unwired: 14 in]
      }
      frame "Action: Get Images" {
        w312 = T15 0 items=["Grayscale (U8)", "Grayscale (I16)", "Grayscale (SGL)", "Complex (CSG)", "RGB (U32)", "HSL (U32)", "RGB (U64)", "Grayscale (U16)"] ("Image Type")
        w315 = T15 0 items=["Grayscale (U8)", "Grayscale (I16)", "Grayscale (SGL)", "Complex (CSG)", "RGB (U32)", "HSL (U32)", "RGB (U64)", "Grayscale (U16)"] ("Image Type")
        w308 = T15 0 items=["Grayscale (U8)", "Grayscale (I16)", "Grayscale (SGL)", "Complex (CSG)", "RGB (U32)", "HSL (U32)", "RGB (U64)", "Grayscale (U16)"] ("Image Type")
        w310 = T15 0 items=["Grayscale (U8)", "Grayscale (I16)", "Grayscale (SGL)", "Complex (CSG)", "RGB (U32)", "HSL (U32)", "RGB (U64)", "Grayscale (U16)"] ("Image Type")
        n133 = call "IMAQ Create"("Image Name"="frogTrace::1", "Image Type"=w310) -> ("New Image"=w305:T3)  [unwired: 3 in, 1 out]
        "frogTrace::1" <- w305
        n134 = call "IMAQ Create"("Image Name"="SpatialImage::1", "Image Type"=w308) -> ("New Image"=w304:T3)  [unwired: 3 in, 1 out]
        "SpatialImage::1" <- w304
        n135 = call "IMAQ Create"("Image Name"="rotated_Spatial", "Image Type"=w312) -> ("New Image"=w302:T3)  [unwired: 3 in, 1 out]
        n136 = call "IMAQ Create"("Image Name"="rotated_Temporal", "Image Type"=w315) -> ("New Image"=w303:T3)  [unwired: 3 in, 1 out]
        n137 = Bundle By Name(cluster=w307, "Images.frogTrace::1"=w305, "Images.SpatialImage::1"=w304, "Images.rotated_Temporal"=w303, "Images.rotated_Spatial"=w302) -> (w306:T10)
        n138 = call <vilib>:"Add State(s) to Queue__jki_lib_state_machine.vi"("State(s) in (\"\")"=w318) -> ("States Out"=w317:string)  [unwired: 14 in]
      }
      frame "Action: User Event Image" {
        n139 = Unbundle By Name(w323) -> ("Images.frogTrace::1"=w322:T3, "Images.SpatialImage::1"=w321:T3, "Images.rotated_Temporal"=w320:T3, "Images.rotated_Spatial"=w319:T3)
        n140 = call "IMAQ Rotate"("Maintain Size"=FALSE, "Angle (degrees)"=sgl 90.0, "Image Dst"=w320, "Image Src"=w322) -> ("error out"=w325:errorcluster, "Image Dst Out"=w334:T3)  [unwired: 6 in]
        "525" <- w334
        n141 = call <vilib>:"Clear Errors.vi"("error in (no error)"=w325) -> ()  [unwired: 5 in, 2 out]
        n142 = call "IMAQ Rotate"("Maintain Size"=FALSE, "Angle (degrees)"=sgl 90.0, "Image Dst"=w319, "Image Src"=w321) -> ("error out"=w328:errorcluster, "Image Dst Out"=w331:T3)  [unwired: 6 in]
        n143 = call "IMAQ Histogram"("Image"=w334) -> ("Histogram Report"=w335:T14)  [unwired: 9 in, 1 out]
        n144 = call <vilib>:"Clear Errors.vi"("error in (no error)"=w328) -> ("error out"=w332:errorcluster)  [unwired: 5 in, 1 out]
        n145 = disable-structure shown="Enabled" {
          disable-tunnel: [w344 w345] -> w333
          disable-tunnel: w332 -> [w343 w346]
          disable-tunnel: w331 -> [w342 w345]
          disable-tunnel: [w340 w346] -> w330
          frame Disabled {
            (unwired) 384.0 ("Target.Y")
            (unwired) 288.0 ("Target.X")
            (unwired) cluster{"xhair size":dbl, "xhair size 2":dbl} {"xhair size"=275.0, "xhair size 2"=275.0} ("size")
            (unwired) u32 16774656 ("Color")
            n146 = call "draw crosshair imaq.vi"("error in (no error)"=w343, "Bounding Rectangle"=T9 {"Left"=0, "Top"=0, "Right"=0, "Bottom"=0}, "image in"=w342) -> ("error out"=w340:errorcluster, "image out"=w344:T3)  [unwired: 7 in]
          }
          frame Enabled {
          }
        }
        "131" <- w333
        "error out" <- w330
        n147 = Unbundle By Name(w335) -> ("Maximal Value"=→"Tank":sgl)
        n148 = call <vilib>:"Add State(s) to Queue__jki_lib_state_machine.vi"("State(s) in (\"\")"=w339) -> ("States Out"=w338:string)  [unwired: 14 in]
      }
    }
  }
  n149 = disable-structure shown="Disabled" {
    frame Disabled {
      n150 = property on="Select device" class="CmbBox" props=["Strings[]"]() -> ()  [unwired: 3 in, 2 out]
    }
    frame Enabled {
    }
  }
